vi "RTS Determine the Correct Defrost.vi"(8 "Error In":errorcluster, 11 "Defrost Info Input":dbl[](array[numeric])) -> (0 "Error Out":errorcluster, 3 "Longest Defrost Cycle data":dbl[](array[numeric]))   [LabVIEW 2016]
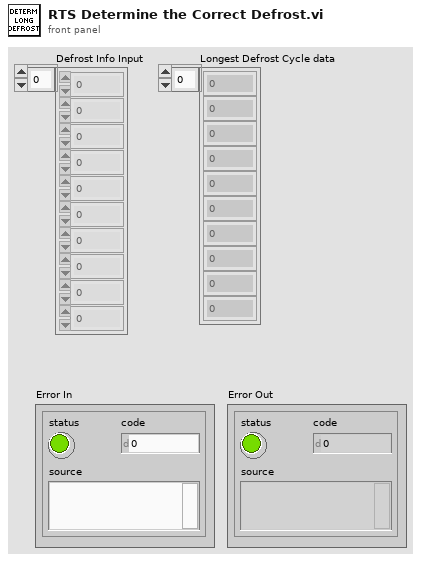
[diagram p1: front panel]
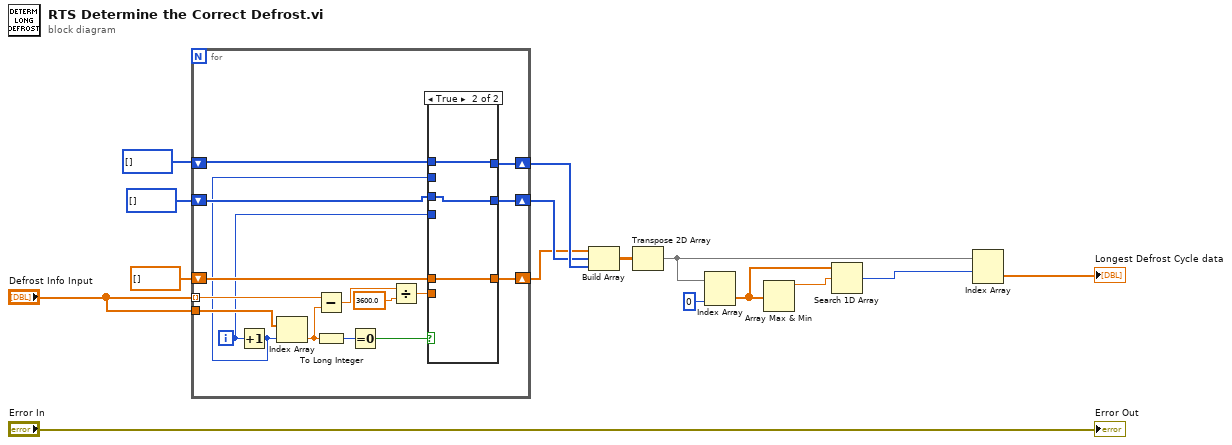
[diagram p0: block diagram]
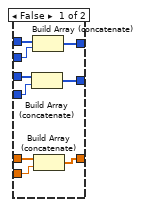
[diagram p2: hidden frame]
diagram:
  n1 = for {
    tunnel: "Defrost Info Input" -> [w31] mode=indexing
    tunnel: "Defrost Info Input" -> [w30]
    shift-right: [w23] -> w5
    shift-left: dbl[] [] -> [w24]
    shift-right: [w20] -> w6
    shift-left: i32[] [] -> [w21]
    shift-right: [w17] -> w7
    shift-left: i32[] [] -> [w18]
    i -> [w19]
    n2 = Increment(x=w19) -> (x+1=w16:i32)
    n3 = Index Array(array=w30, index=w16) -> (element=w27:dbl)
    n4 = Subtract(x=w31, y=w27) -> (x-y=w28:dbl)
    n5 = To Long Integer(number=w27) -> (32bit integer=w26:i32)
    n6 = Equal To 0?(x=w26) -> (x = 0?=w25:bool)
    n7 = Divide(x=w28, y=3600.0) -> (x/y=w22:dbl)
    n8 = case shown="True" w25 {
      tunnel: w24 -> [w40 w43]
      tunnel: [w39 w43] -> w23
      tunnel: w22 -> [w38 _]
      tunnel: w21 -> [w37 w42]
      tunnel: [w36 w42] -> w20
      tunnel: w19 -> [w35 _]
      tunnel: w18 -> [w34 w41]
      tunnel: [w33 w41] -> w17
      tunnel: w16 -> [w32 _]
      frame False {
        n9 = Build Array (concatenate)(w37, w35) -> (w36:i32[])
        n10 = Build Array (concatenate)(w34, w32) -> (w33:i32[])
        n11 = Build Array (concatenate)(w40, w38) -> (w39:dbl[])
      }
      frame True {
      }
    }
  }
  n12 = Build Array(w5, w6, w7) -> (w8:dbl[][])
  n13 = Transpose 2D Array(2D array=w8) -> (transposed array=w12:dbl[][])
  n14 = Index Array(array=w12, index (col)=0 ("disabled index (col)")) -> (element=w11:dbl[])  [unwired: 1 in]
  n15 = Array Max & Min(array=w11) -> (max value=w10:dbl)  [unwired: 3 out]
  n16 = Search 1D Array(1D array=w11, element=w10) -> (index of element=w13:i32)  [unwired: 1 in]
  n17 = Index Array(array=w12, index (row)=w13) -> (element=→"Longest Defrost Cycle data":dbl[])  [unwired: 1 in]
  "Error Out" <- "Error In"
